vi "Rotate.vi"(6 "Synchronication":enum16{"Start", "Wait"}(ring)=enum."Wait", 7 "Description":string, 8 "Command Info In":T1, 9 "Force Degrees":bool, 10 "Turn Direction":string(combo), 11 "Degrees":dbl) -> (0 "Command Info Out":T1)   [LabVIEW 2017]
doc: "This VI notifies the subsystem to perform this command for the given duration, then go back to the default state. Synchronization determines whether this VI Starts the operation and returns immediately, or waits for the operation to complete. The first option is commonly used for TeleOp, and the second for Autonomous sequencing."
uses:
  <vilib>/Rock Robotics/WPI/Framework/Command Status Info.ctl
  <vilib>/Rock Robotics/WPI/Framework/Completion Status.ctl
  <vilib>/Rock Robotics/WPI/Framework/Completion Notifier.ctl
  Implementation/Drive Setpoints.ctl
  Implementation/Drive Operations.ctl
  Framework/Robot Global Data.vi
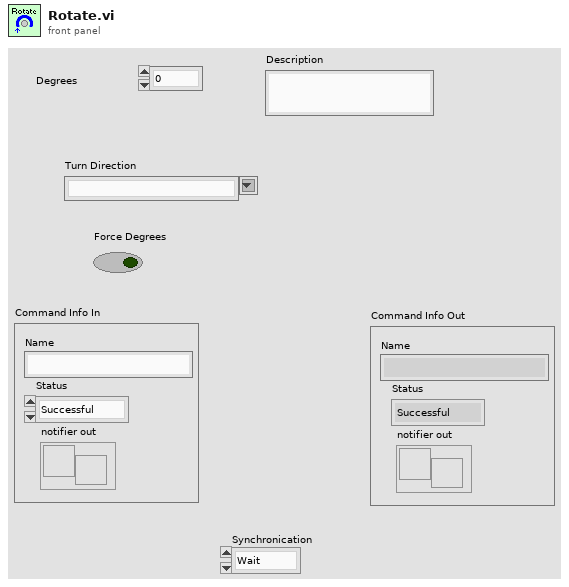
[diagram p1: front panel]
types:
  T1 = typedef "Command Status Info.ctl" = cluster{"Name":string, "Status":T2, "notifier out":T3}
  T2 = typedef "Completion Status.ctl" = enum16{"Successful", "Aborted", "Incomplete"}
  T3 = typedef "Completion Notifier.ctl" = refnum<notifier>
  T4 = typedef "Drive Setpoints.ctl" = cluster{"Operation":T5, "Left Setpoint":dbl, "Right Setpoint":dbl, "Duration":dbl, "Distance (inches)":dbl}
  T5 = typedef "Drive Operations.ctl" = enum16{"Reserve", "Read Current", "Immediate", "Drive for Time", "Drive for Distance", "Rotate"}
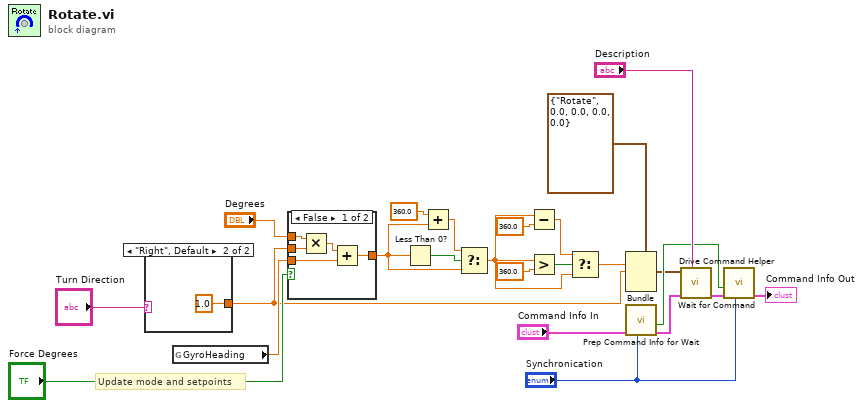
[diagram p0: block diagram]
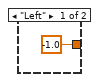
[diagram p2: hidden frame]
diagram:
  # "Update mode and setpoints"
  n1 = case shown="\"Right\", Default" "Turn Direction" {
    tunnel: [-1.0 1.0] -> w12
    frame "Left" {
    }
    frame "Right", Default {
    }
  }
  n2 = global read "Robot Global Data.vi" "GyroHeading"() -> (w14:dbl)
  n3 = case shown="False" "Force Degrees" {
    tunnel: "Degrees" -> [w31 w32]
    tunnel: [w27 w32] -> w10
    tunnel: w14 -> [w28 _]
    tunnel: w12 -> [w30 _]
    frame False {
      n4 = Multiply(x=w31, y=w30) -> (x*y=w29:dbl)
      n5 = Add(x=w29, y=w28) -> (x+y=w27:dbl)
    }
    frame True {
    }
  }
  n6 = Less Than 0?(x=w10) -> (x < 0?=w11:bool)
  n7 = Add(x=360.0, y=w10) -> (x+y=w8:dbl)
  n8 = Select(t=w8, s=w11, f=w10) -> (s? t:f=w5:dbl)
  n9 = Subtract(x=w5, y=360.0) -> (x-y=w3:dbl)
  n10 = Greater?(x=w5, y=360.0) -> (0:w6:bool)
  n11 = Select(t=w3, s=w6, f=w5) -> (s? t:f=w2:dbl)
  n12 = Bundle(cluster=T4 {"Operation"=enum."Rotate", "Left Setpoint"=0.0, "Right Setpoint"=0.0, "Duration"=0.0, "Distance (inches)"=0.0} ("SubSystem Data"), "Left Setpoint"=w2, "Right Setpoint"=w12) -> (w17:T4)  [unwired: 3 in]
  n13 = call <vilib>:"Prep Command Info for Wait.vi"("Synchronication"="Synchronication", "Command Info"="Command Info In") -> ("Command Info"=w21:T1, "Allocated"=w22:bool)  [unwired: 8 in]
  n14 = call "Drive Command Helper.vi"("Description"="Description", "Command Info In"=w21, "SubSystem Data"=w17) -> ("Command Info Out"=w18:T1)  [unwired: 6 in, 2 out]
  n15 = call <vilib>:"Wait for Command.vi"("Synchronication"="Synchronication", "Command Info in"=w18, "Allocated"=w22) -> ("Command Info out"=→"Command Info Out":T1)  [unwired: 8 in]
